vi "18_TimeTaggerNetwork_client.vi"(8 "error in (no error)":errorcluster) -> (0 "error out":errorcluster)   [LabVIEW 2014]
uses:
  SwabianInstruments.TimeTagger
panel:
  out "getOverflowsClient":i64
  out "getOverflows":i64
  out "log messages":string
  out "available servers":string[](array[string])
  out "connected to server":bool
  out "Counter measurement":i32[][](graph)
  in  "stop":bool
  # "With this VI you can connect to a Time Tagger server in your network. First, the VI will scan for available servers and displays the list.\nThe VI will first try to connect to a server on 'localhost', if this does not work, it tries the list of scanned servers.\n\nThe VI performs a Counter measurement on channels 1-4. You can also try to start a server in Python, for example, and connect the client in LabVIEW.\n\nThe VI will also display the return values of the getOverflows() and getOverflowsClient() methods. While overflows on the server may result from insufficient USB transfer or an unlocked SoftwareClock, the client side overflows also include data loss due to insufficient network transfer."
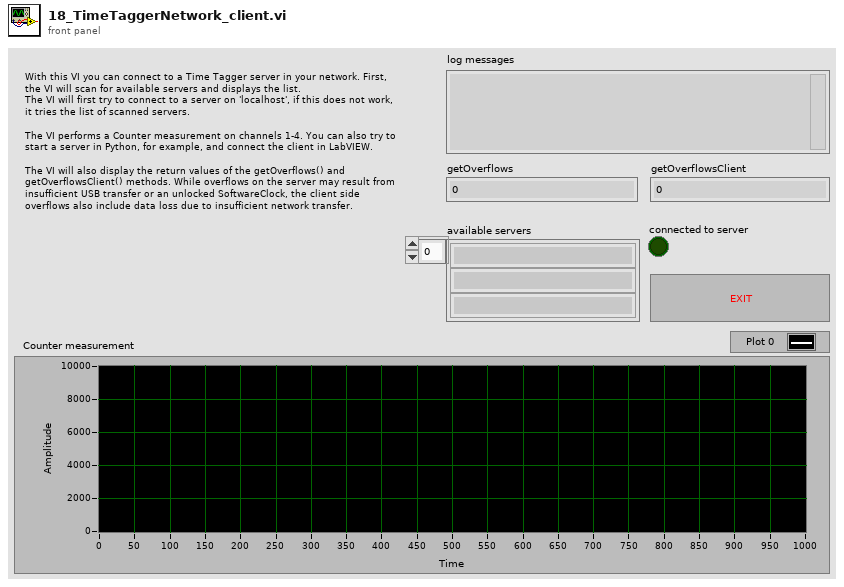
[diagram p1: front panel]
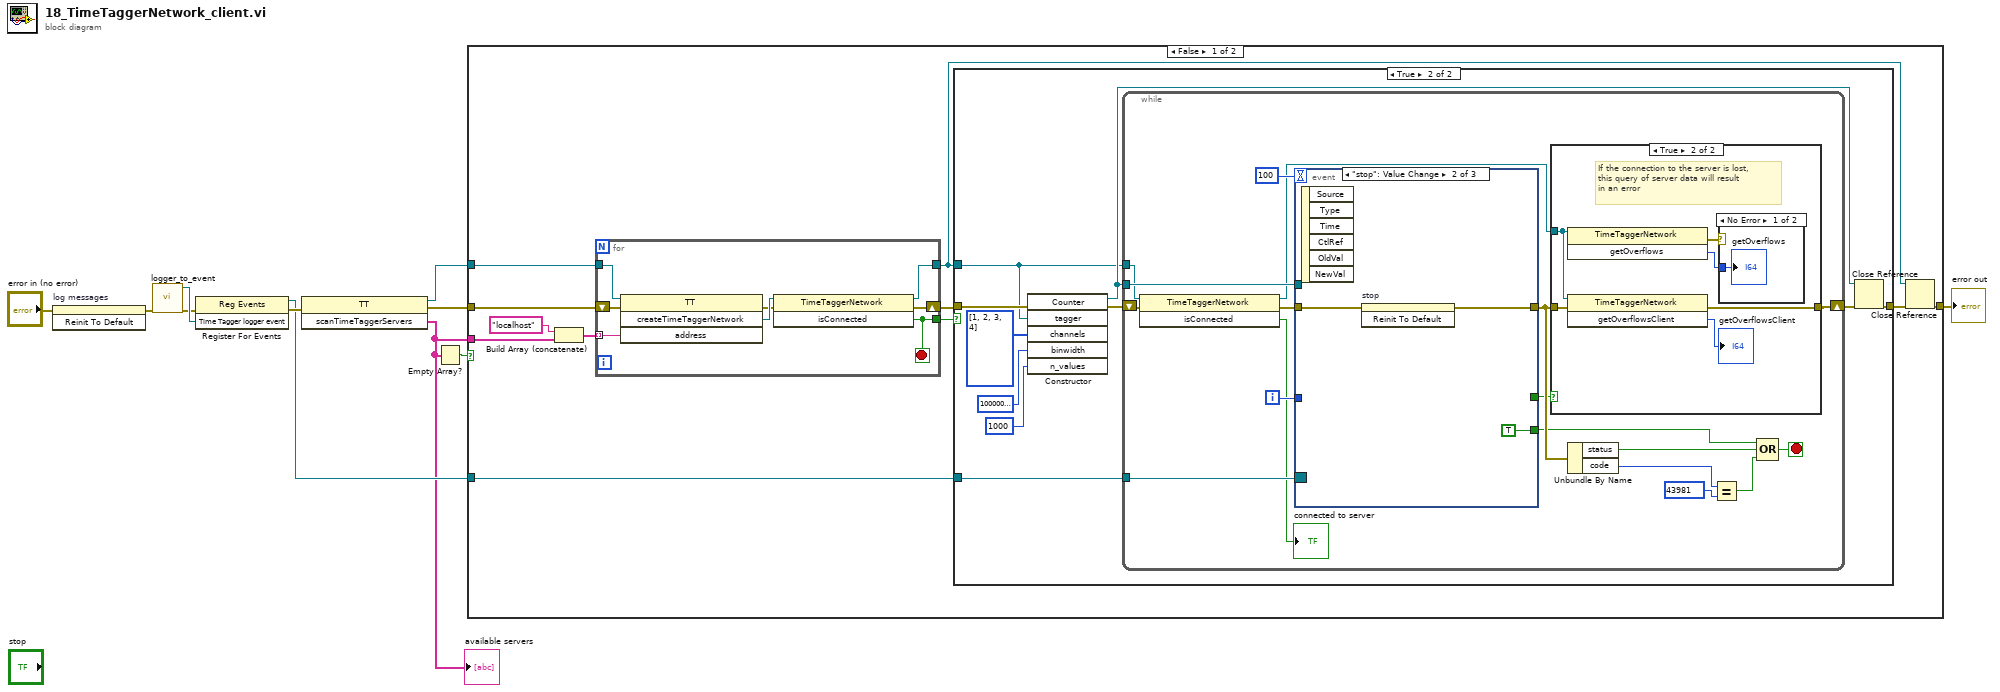
[diagram p0: block diagram]
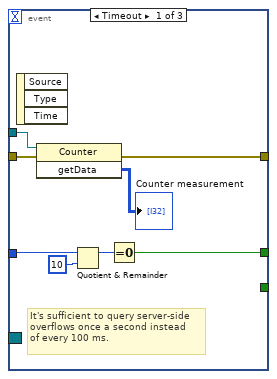
[diagram p5: hidden frame]
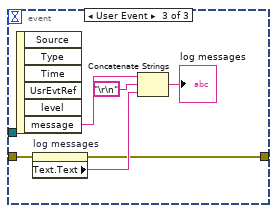
[diagram p6: hidden frame]
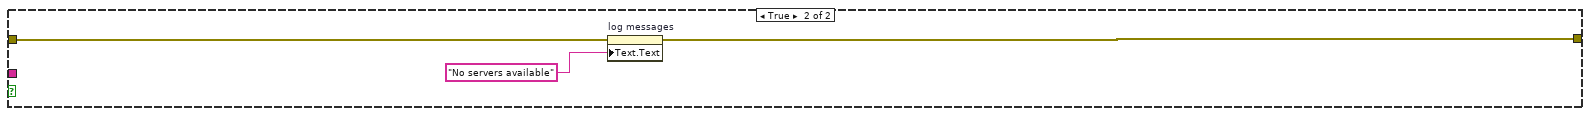
[diagram p7: hidden frame]
diagram:
  n1 = invoke on="log messages" class="Str" method="Reinit To Default"(error in="error in (no error)") -> (error out=w7:errorcluster)  [unwired: 2 in, 2 out]
  n2 = call "logger_to_event.vi"("error in (no error)"=w7) -> ("error out"=w5:errorcluster, "Time Tagger logger event"=w6:refnum<user-event>)  [unwired: 9 in]
  n3 = register-events(error in=w5, w6) -> (reference out=w3:refnum<event-registration>, error out=w4:errorcluster)  [unwired: 1 in]
  n4 = invoke class="TT" method="scanTimeTaggerServers"(error in=w4) -> (reference out=w10:refnum<k24>, error out=w9:errorcluster, "scanTimeTaggerServers"=w1:string[])  [unwired: 2 in]
  "available servers" <- w1
  n5 = Empty Array?(array=w1) -> (empty?=w11:bool)
  n6 = case shown="False" w11 {
    tunnel: w10 -> [w22 _]
    tunnel: [w19 w86] -> w2
    tunnel: w9 -> [w21 w87]
    tunnel: w3 -> [w15 _]
    tunnel: w1 -> [w14 _]
    frame False {
      n7 = Build Array (concatenate)("localhost" ("address"), w14) -> (w12:string[])
      n8 = for {
        tunnel: w22 -> [w30]
        tunnel: [w23] -> w18
        tunnel: [w27] -> w17
        tunnel: w12 -> [w24] mode=indexing
        shift-right: [w25] -> w16
        shift-left: w21 -> [w29]
        stop <- w23 stop-if-true
        n9 = invoke class="TT" method="createTimeTaggerNetwork"(reference=w30, error in=w29, "address"=w24) -> (error out=w26:errorcluster, "createTimeTaggerNetwork"=w28:refnum<k24>)  [unwired: 1 in, 2 out]
        n10 = invoke class="TimeTaggerNetwork" method="isConnected"(reference=w28, error in=w26) -> (reference out=w27:refnum<k24>, error out=w25:errorcluster, "isConnected"=w23:bool)  [unwired: 1 in]
      }
      n11 = case shown="True" w18 {
        tunnel: [w31 w36] -> w20
        tunnel: w17 -> [_ w32]
        tunnel: w16 -> [w31 w35]
        tunnel: w15 -> [_ w33]
        frame False {
        }
        frame True {
          n12 = constructor class="Counter"(error in=w35, "tagger"=w32, "channels"=i32[] [1, 2, 3, 4] ("channel"), "binwidth"=i64 10000000000, "n_values"=1000) -> (reference out=w34:refnum<k24>, error out=w37:errorcluster)  [unwired: 2 in, 5 out]
          n13 = while {
            shift-right: [w49] -> w41
            shift-left: w37 -> [w46]
            tunnel: w34 -> [w59]
            tunnel: w33 -> [w52]
            tunnel: w32 -> [w44]
            i -> [w51]
            stop <- w57 stop-if-true
            n14 = invoke class="TimeTaggerNetwork" method="isConnected"(reference=w44, error in=w46) -> (reference out=w43:refnum<k24>, error out=w45:errorcluster, "isConnected"=→"connected to server":bool)  [unwired: 1 in]
            n15 = event shown="[1] \"stop\": Value Change" {
              selector: w52 -> [_ _ _]
              dyn-events: _ -> [_ _ _]
              timeout: 100 -> [_ _ _]
              tunnel: w45 -> [w74 w78 w84]
              tunnel: [w72 w77 w79] -> w50
              tunnel: w59 -> [w75 _ _]
              tunnel: w51 -> [w71 _ _]
              tunnel: [w68 w76 _] -> w48
              tunnel: [_ w76 _] -> w42
              event Timeout {
                # "It's sufficient to query server-side\noverflows once a second instead\nof every 100 ms."
                n16 = event-data() -> ()  [unwired: 1 in, 3 out]
                n17 = invoke class="Counter" method="getData"(reference=w75, error in=w74) -> (error out=w72:errorcluster, "getData"=→"Counter measurement":i32[][])  [unwired: 1 in, 1 out]
                n18 = Quotient & Remainder(x=w71, y=10) -> (x-y*floor(x/y)=w69:i32)  [unwired: 1 out]
                n19 = Equal To 0?(x=w69) -> (x = 0?=w68:bool)
              }
              event "stop": Value Change {
                w76 = TRUE
                n20 = event-data() -> ()  [unwired: 1 in, 6 out]
                n21 = invoke on="stop" class="Bool" method="Reinit To Default"(error in=w78) -> (error out=w77:errorcluster)  [unwired: 2 in, 2 out]
              }
              event User Event {
                n22 = event-data() -> ("message"=w81:string)  [unwired: 1 in, 5 out]
                n23 = property on="log messages" class="Str"(error in=w84) -> (error out=w79:errorcluster, "Text.Text"=w83:string)  [unwired: 1 in, 1 out]
                n24 = Concatenate Strings(w81, "\r\n", w83) -> (→"log messages":string)
              }
            }
            n25 = case shown="True" w48 {
              tunnel: w43 -> [_ w63]
              tunnel: w50 -> [w60 w61]
              tunnel: [w60 w66] -> w49
              frame False {
              }
              frame True {
                # "If the connection to the server is lost,\nthis query of server data will result\nin an error"
                n26 = invoke class="TimeTaggerNetwork" method="getOverflows"(reference=w63) -> (error out=w62:errorcluster, "getOverflows"=w65:i64)  [unwired: 2 in, 1 out]
                n27 = invoke class="TimeTaggerNetwork" method="getOverflowsClient"(reference=w63, error in=w61) -> (error out=w66:errorcluster, "getOverflowsClient"=→"getOverflowsClient":i64)  [unwired: 1 in, 1 out]
                n28 = case shown="No Error" w62 {
                  tunnel: w65 -> [w67 _]
                  frame No Error {
                    "getOverflows" <- w67
                  }
                  frame Error {
                  }
                }
              }
            }
            n29 = Unbundle By Name(w50) -> ("status"=w56:bool, "code"=w55:i32)
            n30 = Equal?(x=w55, y=43981 ("code")) -> (x = y?=w54:bool)
            n31 = Compound Arithmetic op=OR(w42, w56, w54) -> (w57:bool)
          }
          n32 = Close Reference(reference=w34, error in (no error)=w41) -> (error out=w36:errorcluster)
        }
      }
      n33 = Close Reference(reference=w17, error in (no error)=w20) -> (error out=w19:errorcluster)
    }
    frame True {
      n34 = property on="log messages" class="Str"(error in=w87, "Text.Text"="No servers available") -> (error out=w86:errorcluster)  [unwired: 1 in, 1 out]
    }
  }
  "error out" <- w2
